vi "ReadHemisphereData.vi"(8 "Error in":errorcluster, 10 "Hemisphere Queue Cluster":T1, 11 "VISA UART port":refnum<visa-resource-name>) -> (0 "Error out":errorcluster, 2 "Sentence":string, 3 "Raw string":string)   [LabVIEW 2013]
doc: "This VI takes in Hemisphere data and writes it to the proper queues, which are passed over to HindBrain think for filtering and sending to the notifiers. It is unfinished and untested.\n\nEric Schneider, March 2014"
uses:
  Data/TypeDefs/GPS-Compass Queue Cluster.ctl
  Data/TypeDefs/UTM Location.ctl
panel:
  out "Pitch":dbl
  out "Roll":dbl
  out "Boat Direction":dbl
  out "Boat Speed (m/s)":dbl
  out "Boat Velocity Direction":dbl
  out "Rate of Turn (deg/s)":dbl
  out "Longitude":dbl
  out "Latitude":dbl
  out "Array":string[](array[string])
  in  "time zone":i32
  out "Time":string
  out "NMEA sentences":string
  # "Hemisphere Sense"
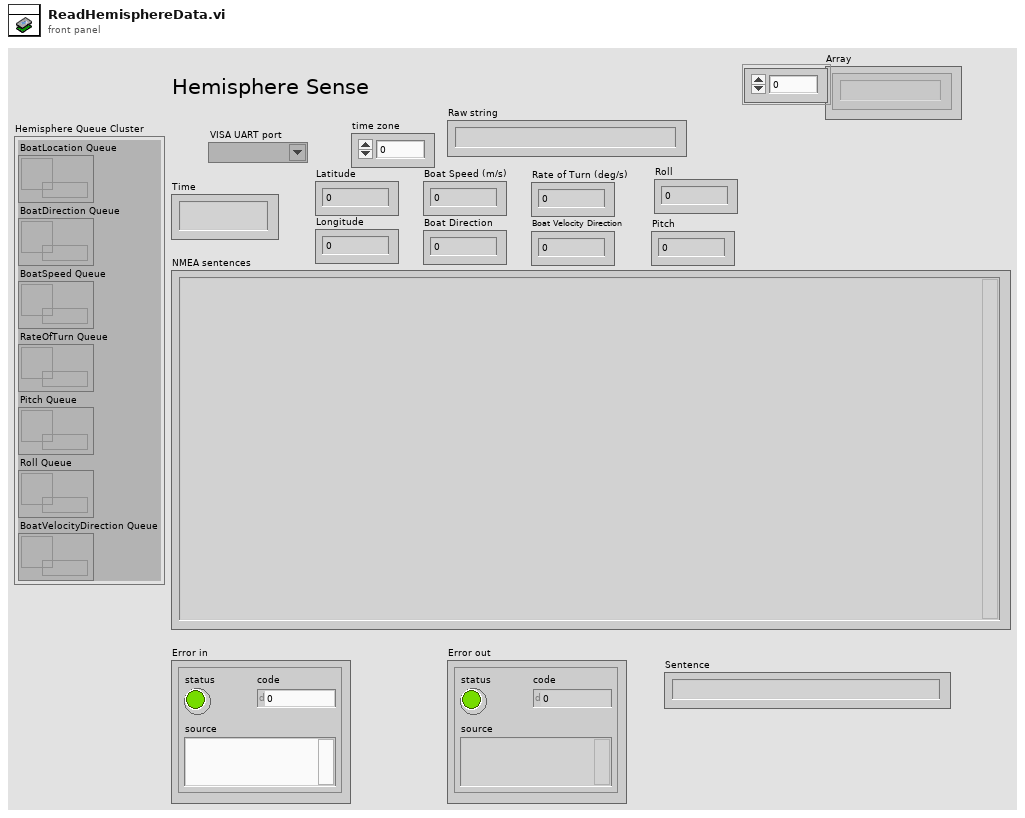
[diagram p1: front panel]
types:
  T1 = typedef "GPS-Compass Queue Cluster.ctl" = cluster{"BoatLocation Queue":refnum<queue>, "BoatDirection Queue":refnum<queue>, "BoatSpeed Queue":refnum<queue>, "RateOfTurn Queue":refnum<queue>, "Pitch Queue":refnum<queue>, "Roll Queue":refnum<queue>, "BoatVelocityDirection Queue ":refnum<queue>}
  T2 = typedef "UTM Location.ctl" = cluster{"UTM Zone":dbl, "Hemisphere":enum16{"North", "South"}, "East":dbl, "North":dbl}
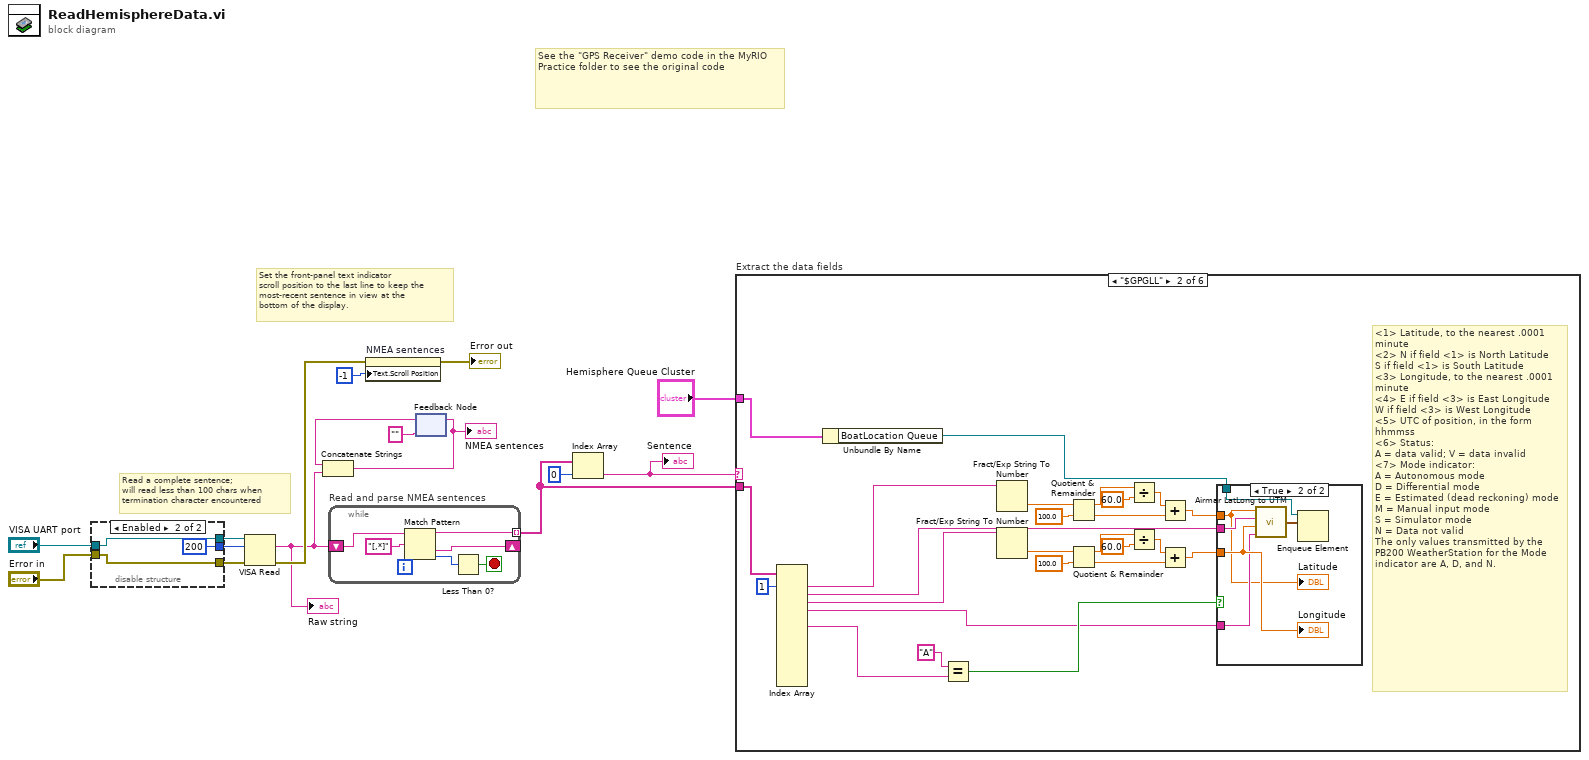
[diagram p0: block diagram]
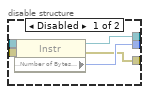
[diagram p2: hidden frame]
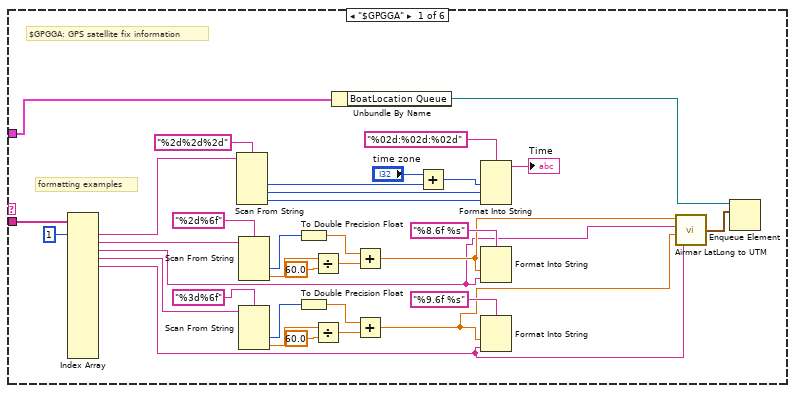
[diagram p3: hidden frame]
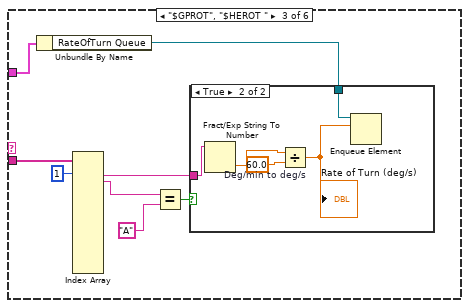
[diagram p5: hidden frame]
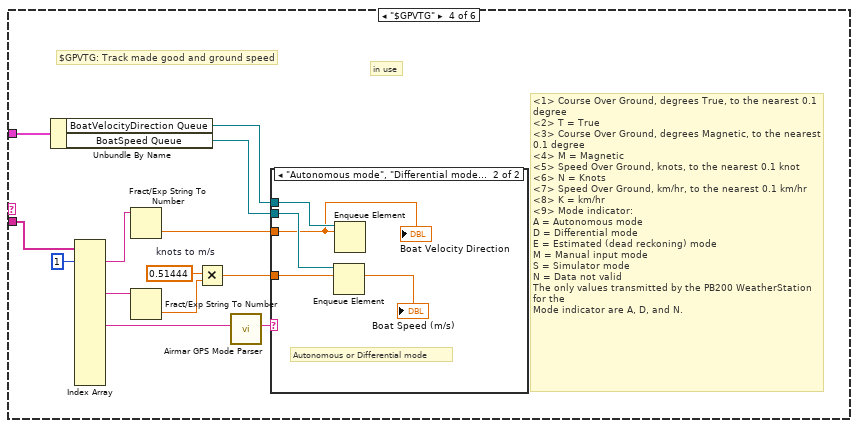
[diagram p7: hidden frame]
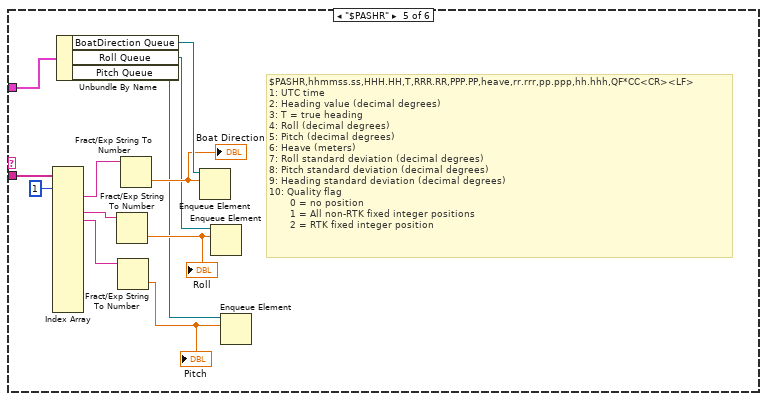
[diagram p9: hidden frame]
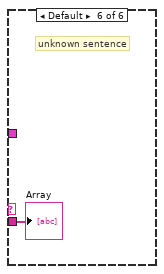
[diagram p10: hidden frame]
diagram:
  # "Set the front-panel text indicator\nscroll position to the last line to keep the\nmost-recent sentence in view at the\nbottom of the display."
  # "Read a complete sentence;\nwill read less than 100 chars when\ntermination character encountered"
  # "See the \"GPS Receiver\" demo code in the MyRIO Practice folder to see the original code"
  n1 = disable-structure shown="Enabled" {
    disable-tunnel: "VISA UART port" -> [w21 w24]
    disable-tunnel: [w20 u32 200 ("Bytes at Port")] -> w5
    disable-tunnel: [w19 w24] -> w4
    disable-tunnel: "Error in" -> [w18 w23]
    disable-tunnel: [w17 w23] -> w2
    frame Disabled {
      n2 = property class="Instr"(reference=w21, error in=w18) -> (reference out=w19:refnum<visa-resource-name>, error out=w17:errorcluster, "Serial Settings:Number of Bytes at Serial Port"=w20:u32)
    }
    frame Enabled {
    }
  }
  n3 = VISA Read(VISA resource name=w4, byte count=w5, error in (no error)=w2) -> (read buffer=w11:string, error out=w16:errorcluster)  [unwired: 2 out]
  "Raw string" <- w11
  n4 = while "Read and parse NMEA sentences" {
    tunnel: [w28] -> w13 mode=indexing
    shift-right: [w27] -> _
    shift-left: w11 -> [w29]
    stop <- w26 stop-if-true
    n5 = Match Pattern(string=w29, regular expression="[,*]") -> (before substring=w28:string, after substring=w27:string, offset past match=w25:i32)  [unwired: 1 in, 1 out]
    n6 = Less Than 0?(x=w25) -> (x < 0?=w26:bool)
  }
  n7 = property on="NMEA sentences" class="Str"(error in=w16, "Text.Scroll Position"=-1) -> (error out=→"Error out":errorcluster)  [unwired: 1 in, 1 out]
  n8 = feedback #1("") -> (w10:string)
  n9 = Concatenate Strings "Concatenate Strings"(w10, w11) -> (w8:string)
  "NMEA sentences" <- w8
  n10 = feedback-in #1(w8) -> ()
  n11 = Index Array "Index Array"(array=w13, index=0) -> (element=w12:string)
  "Sentence" <- w12
  n12 = case "Extract the data fields" shown="\"$GPGLL\"" w12 {
    tunnel: w13 -> [w64 w80 w103 w110 w136 w138]
    tunnel: "Hemisphere Queue Cluster" -> [w37 w81 w100 w109 w135 _]
    frame "$GPGGA" {
      # "formatting examples"
      # "$GPGGA: GPS satellite fix information"
      n13 = Index Array "Index Array"(array=w64, index #1=1 ("index")) -> (element #1=w61:string, element #2=w52:string, element #3=w32:string, element #4=w38:string, element #5=w31:string)  [unwired: 15 in, 11 out]
      n14 = Scan From String "Scan From String"(format string="%2d%2d%2d", input string=w61) -> (output 1=w54:i32, output 2=w57:i32, output 3=w59:i32)  [unwired: 5 in, 3 out]
      n15 = Scan From String(format string="%2d%6f", input string=w52) -> (output 1=w49:i32, output 2=w51:dbl)  [unwired: 4 in, 3 out]
      n16 = Scan From String(format string="%3d%6f", input string=w38) -> (output 1=w42:i32, output 2=w40:dbl)  [unwired: 4 in, 3 out]
      n17 = To Double Precision Float(number=w49) -> (double precision float=w47:dbl)
      n18 = To Double Precision Float(number=w42) -> (double precision float=w44:dbl)
      n19 = Divide(x=w51, y=60.0) -> (x/y=w48:dbl)
      n20 = Divide(x=w40, y=60.0) -> (x/y=w43:dbl)
      n21 = Unbundle By Name(w37) -> ("BoatLocation Queue"=w36:refnum<queue>)
      n22 = Add(x=w47, y=w48) -> (x+y=w34:dbl)
      n23 = Add(x=w44, y=w43) -> (x+y=w33:dbl)
      n24 = Add(x="time zone", y=w54) -> (x+y=w55:i32)
      n25 = Format Into String "Format Into String"(format string="%02d:%02d:%02d", w55, w57, w59) -> (resulting string=→"Time":string)  [unwired: 2 in, 1 out]
      n26 = Format Into String(format string="%8.6f %s", w34, w32) -> ()  [unwired: 2 in, 2 out]
      n27 = Format Into String(format string="%9.6f %s", w33, w31) -> ()  [unwired: 2 in, 2 out]
      n28 = call "Airmar LatLong to UTM.vi"("East/West"=w31, "Longitude"=w33, "North/South"=w32, "Latitude"=w34) -> ("Robot UTM Location"=w35:T2)
      n29 = Enqueue Element(queue=w36, element=w35) -> ()  [unwired: 2 in, 3 out]
    }
    frame "$GPGLL" {
      # "<1> Latitude, to the nearest .0001 minute\n<2> N if field <1> is North Latitude\nS if field <1> is South Latitude\n<3> Longitude, to the nearest .0001 minute\n<4> E if field <3> is East Longitude\nW if field <3> is West Longitude\n<5> UTC of position, in the form hhmmss\n<6> Status:\nA = data valid; V = data invalid\n<7> Mode indicator:\nA = Autonomous mode\nD = Differential mode\nE = Estimated (dead reckoning) mode\nM = Manual input mode\nS = Simulator mode\nN = Data not valid\nThe only values transmitted by the PB200 WeatherStation for the Mode indicator are A, D, and N."
      n30 = Index Array "Index Array"(array=w80, index #1=1 ("index")) -> (element #1=w86:string, element #2=w85:string, element #3=w84:string, element #4=w83:string, element #6=w82:string)  [unwired: 12 in, 8 out]
      n31 = Unbundle By Name(w81) -> ("BoatLocation Queue"=w87:refnum<queue>)
      n32 = Equal?(x="A" ("y"), y=w82) -> (x = y?=w88:bool)
      n33 = Fract/Exp String To Number(string=w86) -> (number=w75:dbl)  [unwired: 3 in, 1 out]
      n34 = Fract/Exp String To Number(string=w84) -> (number=w65:dbl)  [unwired: 3 in, 1 out]
      n35 = Quotient & Remainder(x=w75, y=100.0) -> (x-y*floor(x/y)=w77:dbl, floor(x/y)=w73:dbl)
      n36 = Quotient & Remainder(x=w65, y=100.0) -> (x-y*floor(x/y)=w70:dbl, floor(x/y)=w67:dbl)
      n37 = Divide(x=w77, y=60.0) -> (x/y=w76:dbl)
      n38 = Divide(x=w70, y=60.0) -> (x/y=w69:dbl)
      n39 = Add(x=w76, y=w73) -> (x+y=w74:dbl)
      n40 = Add(x=w69, y=w67) -> (x+y=w68:dbl)
      n41 = case shown="True" w88 {
        tunnel: w85 -> [_ w95]
        tunnel: w68 -> [_ w94]
        tunnel: w83 -> [_ w93]
        tunnel: w87 -> [_ w91]
        tunnel: w74 -> [_ w92]
        frame False {
        }
        frame True {
          n42 = call "Airmar LatLong to UTM.vi"("East/West"=w93, "Longitude"=w94, "North/South"=w95, "Latitude"=w92) -> ("Robot UTM Location"=w90:T2)
          n43 = Enqueue Element(queue=w91, element=w90) -> ()  [unwired: 2 in, 3 out]
          "Latitude" <- w92
          "Longitude" <- w94
        }
      }
    }
    frame "$GPROT", "$HEROT " {
      n44 = Unbundle By Name(w100) -> ("RateOfTurn Queue"=w99:refnum<queue>)
      n45 = Index Array "Index Array"(array=w103, index #1=1 ("index")) -> (element #1=w101:string, element #2=w97:string)  [unwired: 12 in, 11 out]
      n46 = Equal?(x=w97, y="A") -> (x = y?=w96:bool)
      n47 = case shown="True" w96 {
        tunnel: w101 -> [_ w108]
        tunnel: w99 -> [_ w107]
        frame False {
        }
        frame True {
          n48 = Fract/Exp String To Number(string=w108) -> (number=w105:dbl)  [unwired: 3 in, 1 out]
          n49 = Divide "Deg/min to deg/s"(x=w105, y=60.0) -> (x/y=w104:dbl)
          "Rate of Turn (deg/s)" <- w104
          n50 = Enqueue Element(queue=w107, element=w104) -> ()  [unwired: 2 in, 3 out]
        }
      }
    }
    frame "$GPVTG" {
      # "<1> Course Over Ground, degrees True, to the nearest 0.1 degree\n<2> T = True\n<3> Course Over Ground, degrees Magnetic, to the nearest 0.1 degree\n<4> M = Magnetic\n<5> Speed Over Ground, knots, to the nearest 0.1 knot\n<6> N = Knots\n<7> Speed Over Ground, km/hr, to the nearest 0.1 km/hr\n<8> K = km/hr\n<9> Mode indicator:\nA = Autonomous mode\nD = Differential mode\nE = Estimated (dead reckoning) mode\nM = Manual input mode\nS = Simulator mode\nN = Data not valid\nThe only values transmitted by the PB200 WeatherStation for the\nMode indicator are A, D, and N."
      # "in use"
      # "$GPVTG: Track made good and ground speed"
      n51 = Unbundle By Name(w109) -> ("BoatVelocityDirection Queue"=w112:refnum<queue>, "BoatSpeed Queue"=w111:refnum<queue>)
      n52 = Index Array(array=w110, index #1=1 ("index")) -> (element #1=w120:string, element #5=w119:string, element #9=w118:string)  [unwired: 15 in, 13 out]
      n53 = Fract/Exp String To Number(string=w120) -> (number=w117:dbl)  [unwired: 3 in, 1 out]
      n54 = Fract/Exp String To Number(string=w119) -> (number=w115:dbl)  [unwired: 3 in, 1 out]
      n55 = Multiply "knots to m/s"(x=0.51444 ("y"), y=w115) -> (x*y=w116:dbl)
      n56 = call "Airmar GPS Mode Parser.vi"("GPS Mode (Char)"=w118) -> ("GPS Mode (Description)"=w113:string)  [unwired: 6 in]
      n57 = case shown="\"Autonomous mode\", \"Differential mode\"" w113 {
        tunnel: w117 -> [_ w123]
        tunnel: w116 -> [_ w122]
        tunnel: w112 -> [_ w125]
        tunnel: w111 -> [_ w124]
        frame "Data not valid", Default {
          # "Data not valid"
        }
        frame "Autonomous mode", "Differential mode" {
          # "Autonomous or Differential mode"
          n58 = Enqueue Element(queue=w124, element=w122) -> ()  [unwired: 2 in, 3 out]
          n59 = Enqueue Element(queue=w125, element=w123) -> ()  [unwired: 2 in, 3 out]
          "Boat Velocity Direction" <- w123
          "Boat Speed (m/s)" <- w122
        }
      }
    }
    frame "$PASHR" {
      # "$PASHR,hhmmss.ss,HHH.HH,T,RRR.RR,PPP.PP,heave,rr.rrr,pp.ppp,hh.hhh,QF*CC<CR><LF>\n1: UTC time\n2: Heading value (decimal degrees)\n3: T = true heading\n4: Roll (decimal degrees)\n5: Pitch (decimal degrees)\n6: Heave (meters)\n7: Roll standard deviation (decimal degrees)\n8: Pitch standard deviation (decimal degrees)\n9: Heading standard deviation (decimal degrees)\n10: Quality flag\n       0 = no position\n       1 = All non-RTK fixed integer positions\n       2 = RTK fixed integer position"
      n60 = Index Array(array=w136, index #1=1 ("index")) -> (element #2=w133:string, element #4=w128:string, element #5=w127:string)  [unwired: 15 in, 13 out]
      n61 = Unbundle By Name(w135) -> ("BoatDirection Queue"=w134:refnum<queue>, "Roll Queue"=w130:refnum<queue>, "Pitch Queue"=w129:refnum<queue>)
      n62 = Fract/Exp String To Number(string=w128) -> (number=w131:dbl)  [unwired: 3 in, 1 out]
      "Roll" <- w131
      n63 = Fract/Exp String To Number(string=w127) -> (number=w126:dbl)  [unwired: 3 in, 1 out]
      "Pitch" <- w126
      n64 = Fract/Exp String To Number(string=w133) -> (number=w132:dbl)  [unwired: 3 in, 1 out]
      "Boat Direction" <- w132
      n65 = Enqueue Element(queue=w134, element=w132) -> ()  [unwired: 2 in, 3 out]
      n66 = Enqueue Element(queue=w130, element=w131) -> ()  [unwired: 2 in, 3 out]
      n67 = Enqueue Element(queue=w129, element=w126) -> ()  [unwired: 2 in, 3 out]
    }
    frame Default {
      # "unknown sentence"
      "Array" <- w138
    }
  }
